vi "Issue Software Trigger.vi"(8 "error in (no error)":errorcluster, 11 "TLCamera Reference":refnum<k24>) -> (0 "error out":errorcluster, 3 "TLCamera reference out":refnum<k24>)   [LabVIEW 2020]
uses:
  C:/GEECS/Developers Version/source/Device Drivers/Point Grey Camera/Library_X86/Thorlabs.TSI.TLCameraInterfaces.dll
  Point Grey Camera/Library_X86/Thorlabs.TSI.TLCameraInterfaces.dll
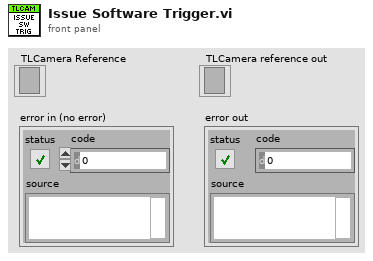
[diagram p1: front panel]
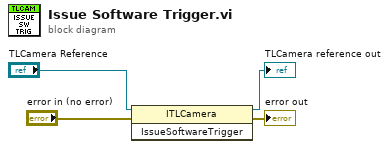
[diagram p0: block diagram]
diagram:
  n1 = invoke class="ITLCamera" method="IssueSoftwareTrigger"(reference="TLCamera Reference", error in="error in (no error)") -> (reference out=→"TLCamera reference out":refnum<k24>, error out=→"error out":errorcluster)  [unwired: 1 in, 1 out]
